vi "Controller Request Stop.vi"(7 "Sync Objects":T3, 8 "error in (no error)":errorcluster) -> (0 "error out":errorcluster)   [LabVIEW 2011, in "Controller VIs.lvlib"]
doc: "Requests the completion of all parallel loops running in the FOFB Controller. Sends a stop notification through the \"Stop Notifier\" and forces all blocking notifiers to be released."
uses:
  Controller VIs.lvlib
  Types Definitions/Type Synchronization Objects.ctl
  Types Definitions/Type Blocking Synchronization Objects.ctl
  Types Definitions/Type FA Request Parameters.ctl
  Types Definitions/Type BPM and PS select cluster.ctl
  Types Definitions/Type FA File Parameters.ctl
  Types Definitions/Type Monitoring Data.ctl
  Types Definitions/Type Diagnostics Data.ctl
  Types Definitions/Type CPU Loads Array.ctl
  Types Definitions/Type CPU Loads.ctl
  Types Definitions/Type Non-blocking Synchronization Objects.ctl
  Types Definitions/Type FOFB Variables.ctl
  Types Definitions/Type Actuation State.ctl
  Misc VIs.lvlib
  Type Definitions.lvlib
panel:
  out "Blocking":T1
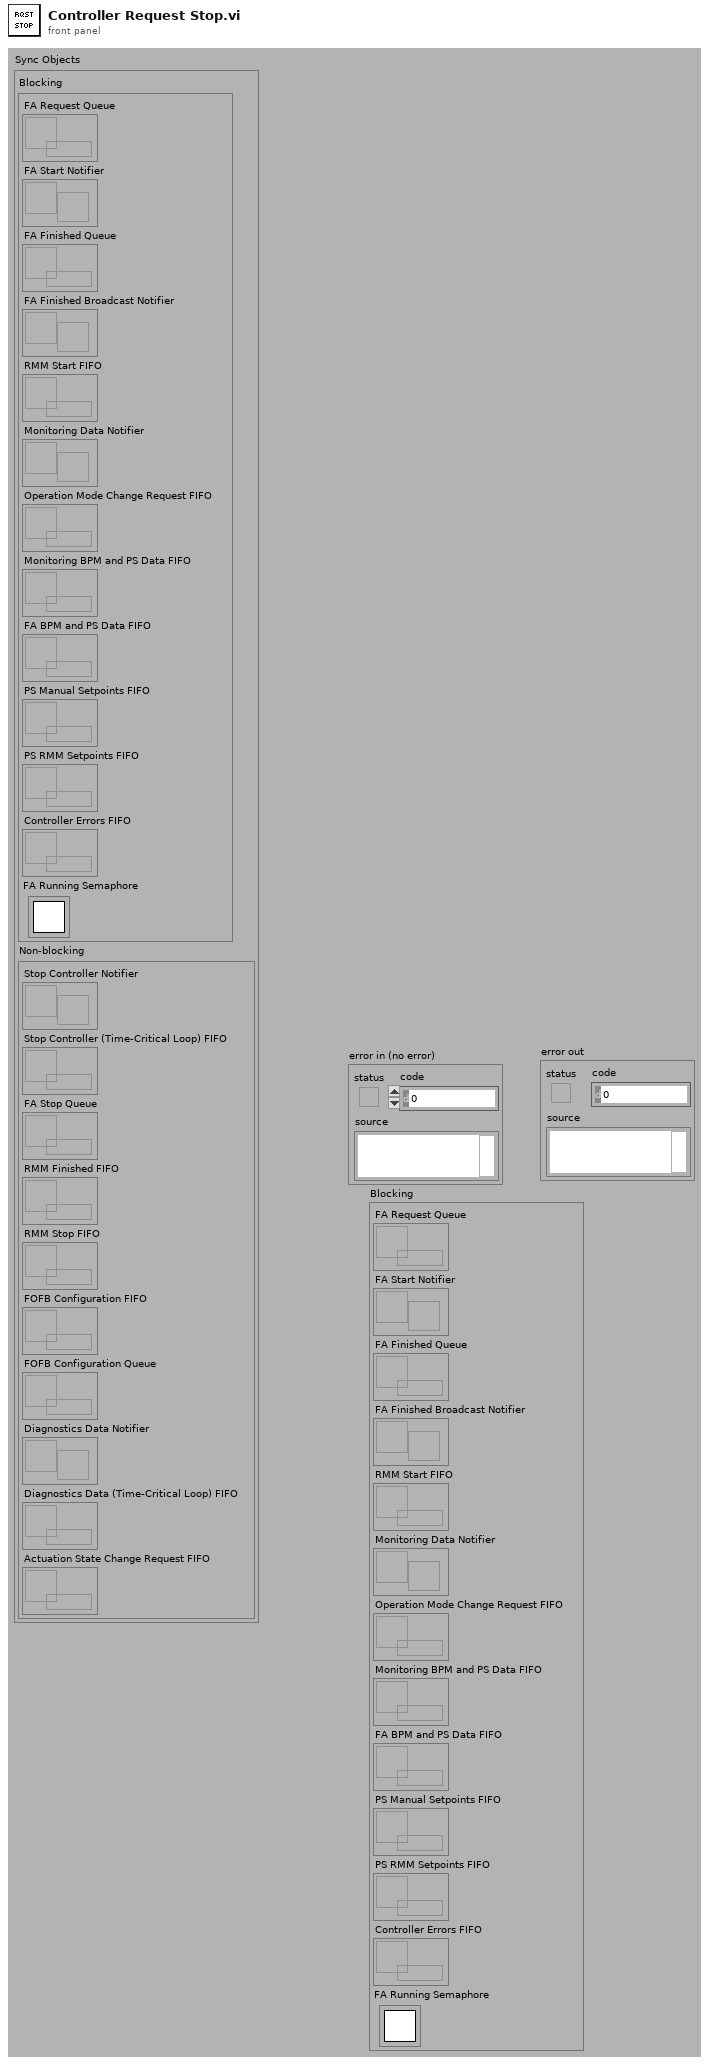
[diagram p1: front panel]
types:
  T1 = typedef "Type Definitions.lvlib/Type Blocking Synchronization Objects.ctl" = cluster{"FA Request Queue":refnum<queue>, "FA Start Notifier":refnum<notifier>, "FA Finished Queue":refnum<queue>, "FA Finished Broadcast Notifier":refnum<notifier>, "RMM Start FIFO":refnum<k33>, "Monitoring Data Notifier":refnum<notifier>, "Operation Mode Change Request FIFO":refnum<k33>, "Monitoring BPM and PS Data FIFO":refnum<k33>, "FA BPM and PS Data FIFO":refnum<k33>, "PS Manual Setpoints FIFO":refnum<k33>, "PS RMM Setpoints FIFO":refnum<k33>, "Controller Errors FIFO":refnum<k33>, "FA Running Semaphore":T2}
  T2 = typedef "Semaphore RefNum" = refnum<k1>
  T3 = typedef "Type Definitions.lvlib/Type Synchronization Objects.ctl" = cluster{"Blocking":T1, "Non-blocking":T4}
  T4 = typedef "Type Definitions.lvlib/Type Non-blocking Synchronization Objects.ctl" = cluster{"Stop Controller Notifier":refnum<notifier>, "Stop Controller (Time-Critical Loop) FIFO":refnum<k33>, "FA Stop Queue":refnum<queue>, "RMM Finished FIFO":refnum<k33>, "RMM Stop FIFO":refnum<k33>, "FOFB Configuration FIFO":refnum<k33>, "FOFB Configuration Queue":refnum<queue>, "Diagnostics Data Notifier":refnum<notifier>, "Diagnostics Data (Time-Critical Loop) FIFO":refnum<k33>, "Actuation State Change Request FIFO":refnum<k33>}
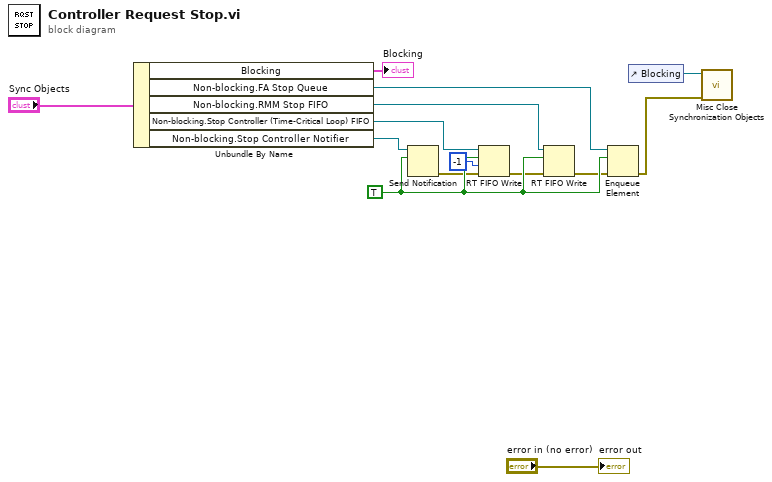
[diagram p0: block diagram]
diagram:
  w7 = TRUE ("notification")
  n1 = Unbundle By Name("Sync Objects") -> ("Blocking"=→"Blocking":T1, "Non-blocking.FA Stop Queue"=w13:refnum<queue>, "Non-blocking.RMM Stop FIFO"=w12:refnum<k33>, "Non-blocking.Stop Controller (Time-Critical Loop) FIFO"=w9:refnum<k33>, "Non-blocking.Stop Controller Notifier"=w11:refnum<notifier>)
  n2 = Send Notification(notification=w7, notifier=w11) -> (error out=w1:errorcluster)  [unwired: 1 in, 1 out]
  n3 = RT FIFO Write(0:w9, 1:w7, 2:-1 ("timeout in ms (0)"), 3:w1) -> (11:w2:errorcluster)  [unwired: 1 in, 3 out]
  n4 = RT FIFO Write(0:w12, 1:w7, 3:w2) -> (11:w3:errorcluster)  [unwired: 2 in, 3 out]
  n5 = Enqueue Element(queue=w13, element=w7, error in (no error)=w3) -> (error out=w4:errorcluster)  [unwired: 1 in, 2 out]
  n6 = control-ref of="Blocking"() -> (w5:refnum<vi>)
  n7 = call "Misc Close Synchronization Objects.vi"("error in (no error)"=w4, "Cluster Reference"=w5) -> ()  [unwired: 9 in, 1 out]
  "error out" <- "error in (no error)"
